vi "Select Channels.vi"(8 "error in (no error)":errorcluster, 11 "Node Ptr":u64 format="%.0x") -> (0 "error out":errorcluster)   [LabVIEW 2015, in "Protection and Rolling Counter Addon System Explorer.lvlib"]
uses:
  Protection and Rolling Counter Addon System Explorer.lvlib
  Shared/SubVIs/GUID Lookup.vi
  <vilib>/NI Veristand/Custom Device API/Custom Device API.lvlib
  Shared/Protection and Rolling Counter Addon Shared.lvlib
panel:
  in  "Tag":string
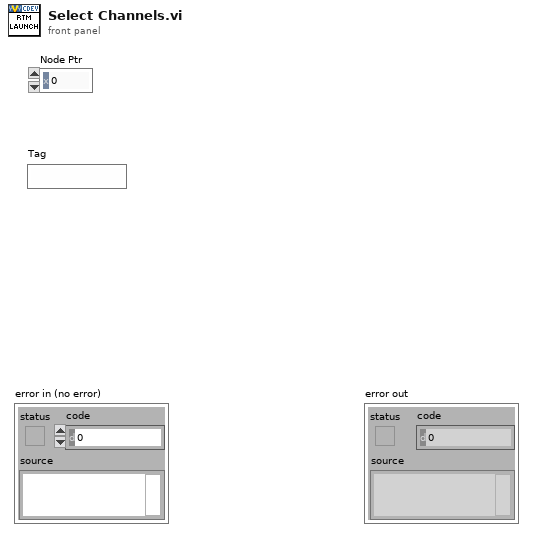
[diagram p1: front panel]
types:
  T1 = typedef "Custom Device API.lvlib/Custom Device Item Ref.ctl" = u64
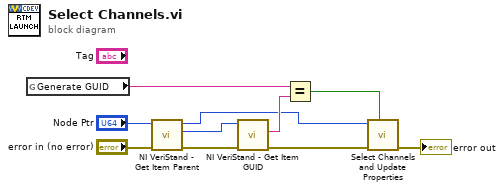
[diagram p0: block diagram]
diagram:
  n1 = global read "GUID Lookup.vi" "Generate GUID"() -> (w6:string)
  n2 = call <vilib>:"NI VeriStand - Get Item Parent.vi"("error in (no error)"="error in (no error)", "Item Ref in"="Node Ptr") -> ("error out"=w2:errorcluster, "Parent Ref"=w4:T1, "Item Ref out"=w1:T1)  [unwired: 6 in, 1 out]
  n3 = call <vilib>:"NI VeriStand - Get Item GUID.vi"("error in (no error)"=w2, "Item Ref in"=w4) -> ("error out"=w8:errorcluster, "GUID"=w9:string)  [unwired: 7 in, 1 out]
  n4 = Equal?(x=w6, y=w9) -> (x = y?=w5:bool)
  n5 = call "Select Channels and Update Properties.vi"("Generate?"=w5, "error in (no error)"=w8, "Node Ptr"=w1) -> ("error out"=→"error out":errorcluster)  [unwired: 8 in]
